vi "SetWindowMouseGrab.vi"(8 "No Error":errorcluster, 10 "Grabbed":bool, 11 "Window [SDL_Window *]":i64 format="%.0x") -> (0 "Error Out":errorcluster)   [LabVIEW 2024, in "SDL3.lvlib" / "Video.lvlib"]
doc: "<B>Summary</B>\nSet a window's mouse grab mode.\n\n<B>Remarks</B>\nMouse grab confines the mouse cursor to the window."
uses:
  Video.lvlib
  Lib/Win32/SDL3.dll
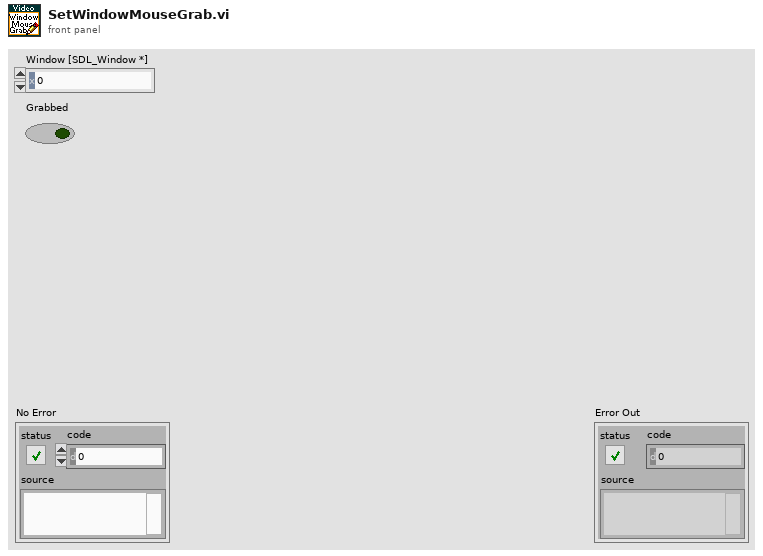
[diagram p1: front panel]
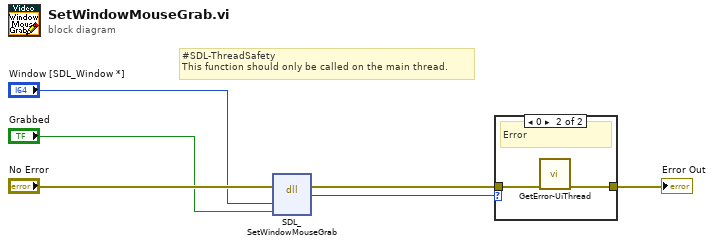
[diagram p0: block diagram]
diagram:
  # "#SDL-ThreadSafety\nThis function should only be called on the main thread."
  n1 = dll-call lib="C:/Users/Thomas/Documents/Projects/LV-SDL3/Lib/Win32/SDL3.dll" fn="SDL_SetWindowMouseGrab"(error in="No Error", "window"="Window [SDL_Window *]", "grabbed"="Grabbed") -> (error out=w3:errorcluster, "return type"=w2:i32)  [unwired: 4 in, 1 out]
  n2 = case shown="0" w2 {
    tunnel: w3 -> [w7 w9]
    tunnel: [w7 w8] -> w5
    frame Default {
      # "Ok"
    }
    frame 0 {
      # "Error"
      n3 = call "GetError-UiThread.vi"("No Error"=w9) -> ("error out"=w8:errorcluster)  [unwired: 10 in]
    }
  }
  "Error Out" <- w5
